vi "Initialize.vi"(8 "error in (no error)":errorcluster, 9 "Parameters In":variant, 10 "Name":string) -> (0 "error out":errorcluster, 3 "Sequence out":refnum<class "Sequence.lvclass">)   [LabVIEW 2015, in "Mediator.lvlib" / "Sequence.lvclass"]
doc: "This creates a new sequence"
uses:
  Sequence.lvclass
  Sequence.lvclass/Sequence.ctl
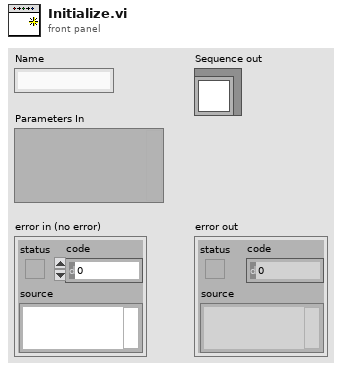
[diagram p1: front panel]
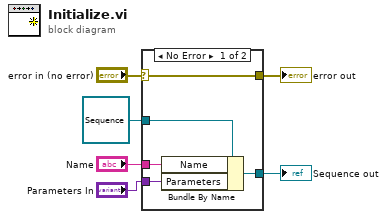
[diagram p0: block diagram]
diagram:
  n1 = case shown="No Error" "error in (no error)" {
    selector: "error in (no error)" -> [w11 w13]
    tunnel: [w11 w13] -> w5
    tunnel: [w9 w12] -> w3
    tunnel: refnum<class "Sequence.lvclass"> refnum ("Sequence in") -> [w10 w12]
    tunnel: "Name" -> [w8 _]
    tunnel: "Parameters In" -> [w7 _]
    frame No Error {
      n2 = Bundle By Name(cluster=w10, "Name"=w8, "Parameters"=w7) -> (w9:refnum<class "Sequence.lvclass">)
    }
    frame Error {
    }
  }
  "error out" <- w5
  "Sequence out" <- w3
